vi "Num to BCD.vi"(11 "Numeric":i32) -> (3 "BCD":u8 format="%.0x")   [LabVIEW 2018]
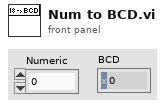
[diagram p1: front panel]
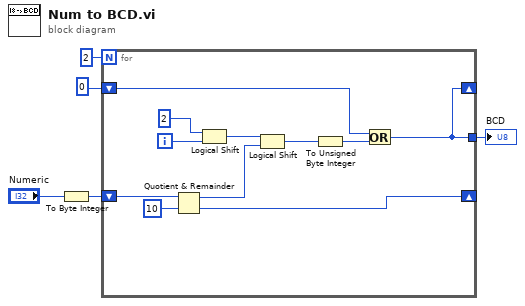
[diagram p0: block diagram]
diagram:
  n1 = To Byte Integer(number="Numeric") -> (8bit integer=w2:i8)
  n2 = for {
    N: 2 -> [_]
    shift-right: [w7] -> _
    shift-left: u8 0 -> [w8]
    shift-right: [w6] -> _
    shift-left: w2 -> [w13]
    tunnel: [w7] -> w3
    i -> [w16]
    n3 = Quotient & Remainder(x=w13, y=i8 10) -> (x-y*floor(x/y)=w11:i8, floor(x/y)=w6:i8)
    n4 = Logical Shift(y=i16 2, x=w16) -> (x << y=w14:i32)
    n5 = Logical Shift(y=w14, x=w11) -> (x << y=w10:i8)
    n6 = To Unsigned Byte Integer(number=w10) -> (unsigned 8bit integer=w9:u8)
    n7 = Or(x=w8, y=w9) -> (x .or. y?=w7:u8)
  }
  "BCD" <- w3
